vi "Set_Sensor_Units.vi"(1 "Weather sensor units":T1 {"Elevation" items=["m", "feet"]; "Wind speed unit" items=["mile/hour", "nots", "km/hour", "m/s"]; "Pressure unit" items=["inch", "mm", "mbar", "hPascal"]; "Rain fall unit" items=["inches", "mm"]; "Temperature unit" items=["Fahrenheit", "Celcius"]}) -> (0 "Succes?":bool)   [LabVIEW 2012]
uses:
  VantagePro.dll
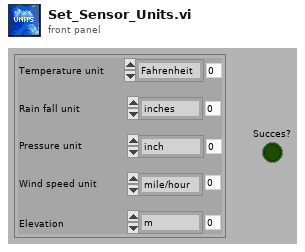
[diagram p1: front panel]
types:
  T1 = cluster{"Temperature unit":i8, "Rain fall unit":i8, "Pressure unit":i8, "Wind speed unit":i8, "Elevation":i8}
  T2 = cluster{"TempUnit":i8, "RainUnit":i8, "PressUnit":i8, "WindUnit":i8, "ElevUnit":i8}
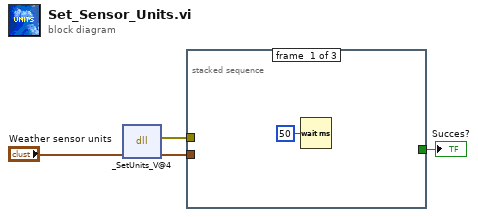
[diagram p0: block diagram]
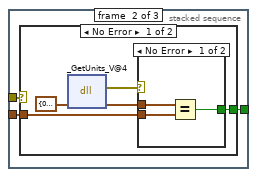
[diagram p2: hidden frame]
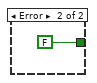
[diagram p3: hidden frame]
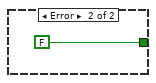
[diagram p4: hidden frame]
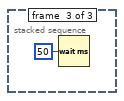
[diagram p5: hidden frame]
diagram:
  n1 = dll-call lib="C:/Users/Bob van Eijk/Desktop/LabView Projects 12/HiSPARC Weather Station/Develop/VantagePro.dll" fn="_SetUnits_V@4" label="Call Library Function\nSet Weather Units"("WeatherUnits"="Weather sensor units") -> (error out=w1:errorcluster, "WeatherUnits"=w2:T1)  [unwired: 3 in, 2 out]
  n2 = stacked-sequence {
    tunnel: [_ w8 _] -> w4
    tunnel: w2 -> [_ w7 _]
    tunnel: w1 -> [_ w6 _]
    frame #0 {
      n3 = Wait (ms)(milliseconds to wait=u32 50) -> ()  [unwired: 1 out]
    }
    frame #1 {
      n4 = case shown="No Error" w6 {
        tunnel: w7 -> [w13 _]
        tunnel: [w12 FALSE] -> w8
        frame No Error {
          n5 = dll-call lib="C:/Users/Bob van Eijk/Desktop/LabView Projects 12/HiSPARC Weather Station/Develop/VantagePro.dll" fn="_GetUnits_V@4" label="Call Library Function\nGet Units"("WeatherUnits"=T2 {"TempUnit"=0, "RainUnit"=0, "PressUnit"=0, "WindUnit"=0, "ElevUnit"=0} ("Weather units")) -> (error out=w9:errorcluster, "WeatherUnits"=w11:T2)  [unwired: 3 in, 2 out]
          n6 = case shown="No Error" w9 {
            tunnel: w13 -> [w16 _]
            tunnel: [w15 FALSE] -> w12
            tunnel: w11 -> [w14 _]
            frame No Error {
              n7 = Equal?(x=w14, y=w16) -> (x = y?=w15:bool)
            }
            frame Error {
            }
          }
        }
        frame Error {
        }
      }
    }
    frame #2 {
      n8 = Wait (ms)(milliseconds to wait=u32 50) -> ()  [unwired: 1 out]
    }
  }
  "Succes?" <- w4
